vi "Busy Bar.vi"(9 "basetime":timestamp, 10 "ms wait (200)":i32=200) -> (1 "Elapsed Seconds":dbl, 2 "Time":string, 3 "Busy Bar":bool[](array[boolean])=[FALSE, FALSE, FALSE, TRUE, FALSE, FALSE, FALSE, TRUE, FALSE, FALSE, FALSE, TRUE, FALSE, FALSE, FALSE, TRUE, FALSE, FALSE, FALSE, TRUE, FALSE, FALSE, FALSE, TRUE, FALSE, FALSE, FALSE, TRUE, FALSE, FALSE, FALSE, TRUE])   [LabVIEW 2017]
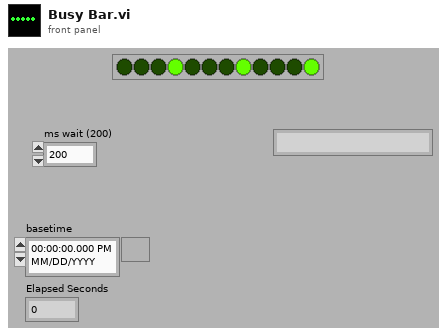
[diagram p1: front panel]
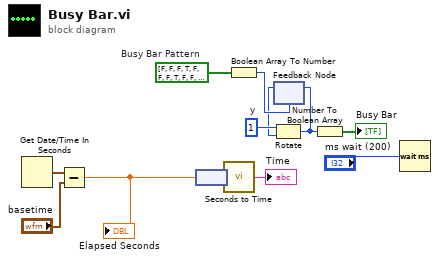
[diagram p0: block diagram]
diagram:
  w7 = bool[] [FALSE, FALSE, FALSE, TRUE, FALSE, FALSE, FALSE, TRUE, FALSE, FALSE, FALSE, TRUE, FALSE, FALSE, FALSE, TRUE, FALSE, FALSE, FALSE, TRUE, FALSE, FALSE, FALSE, TRUE, FALSE, FALSE, FALSE, TRUE, FALSE, FALSE, FALSE, TRUE]  # Busy Bar Pattern
  w9 = u32 1  # y
  n1 = Get Date/Time In Seconds() -> (seconds since 1Jan1904=w4:timestamp)
  n2 = Subtract(x=w4, y="basetime") -> (x-y=w5:dbl)
  "Elapsed Seconds" <- w5
  n3 = node(w5) -> (w1:dbl[unit])
  n4 = call "Seconds to Time.vi"("Seconds"=w1) -> ("Time"=→"Time":string)
  n5 = Boolean Array To Number(Boolean array=w7) -> (number=w12:u32)
  n6 = feedback #1(w12) -> (w8:u32)
  n7 = Rotate(1:w8, 2:w9) -> (0:w11:u32)
  n8 = feedback-in #1(w11) -> ()
  n9 = Number To Boolean Array(number=w11) -> (Boolean array=→"Busy Bar":bool[])
  n10 = Wait (ms)(milliseconds to wait="ms wait (200)") -> ()  [unwired: 1 out]
